vi "gearedMotorPosControl (SubVI).vi"(6 "Reset":bool, 8 "error in (no error)":errorcluster, 9 "PID gains":T1={"proportional gain (Kc)"=2.0, "integral time (Ti, min)"=0.01, "derivative time (Td, min)"=0.00010000000000000003}, 10 "Position (deg)":dbl, 11 "dt":i64) -> (0 "error out":errorcluster, 1 "Waveform Chart":T2(graph), 2 "MotorEncoder (deg)":dbl)   [LabVIEW 2019, in "SJCube.lvlib"]
uses:
  SJCube.lvlib
  <vilib>/addons/control/pid/NI_PID_pid.lvlib
  <vilib>/addons/control/pid/pid.llb/PID (DBL).vi
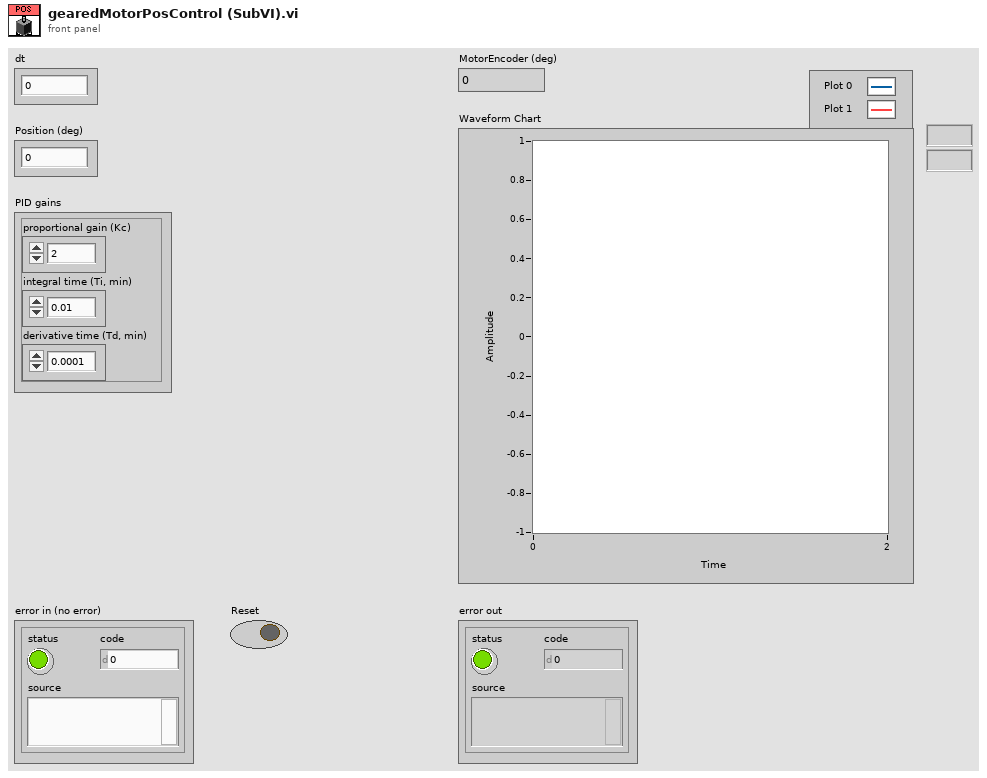
[diagram p1: front panel]
types:
  T1 = cluster{"proportional gain (Kc)":dbl, "integral time (Ti, min)":dbl, "derivative time (Td, min)":dbl}
  T2 = cluster{"Position (deg)":dbl, "MotorEncoder (deg)":dbl}
  T3 = cluster{"Position (deg)":dbl, "gearedMotorEncoder (deg)":dbl}
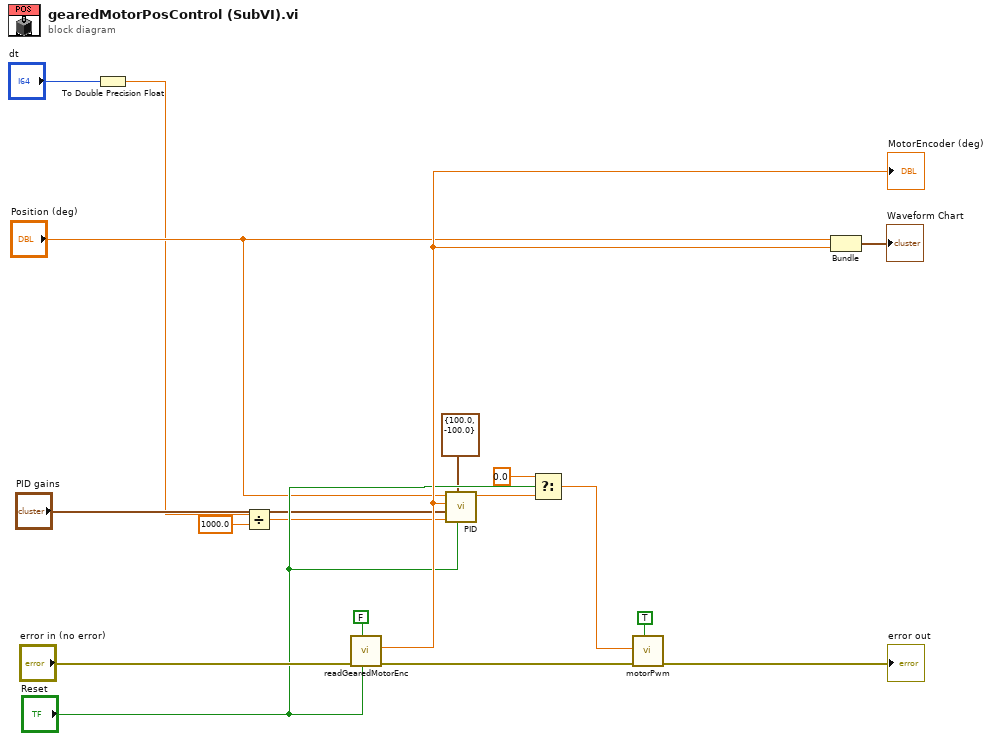
[diagram p0: block diagram]
diagram:
  n1 = To Double Precision Float(number="dt") -> (double precision float=w3:dbl)
  n2 = Divide(x=w3, y=1000.0) -> (x/y=w1:dbl)
  n3 = call "readGearedMotorEnc.vi"("Reset Counter"="Reset", "Reverse ENC?"=FALSE, "error in (no error)"="error in (no error)") -> ("error out"=w10:errorcluster, "gearedMotorEncoder (deg)"=w16:dbl)  [unwired: 7 in]
  "MotorEncoder (deg)" <- w16
  n4 = call-poly <vilib>:"PID.vi"("reinitialize? (F)"="Reset", "output range"=cluster{"output high":dbl, "output low":dbl} {"output high"=100.0, "output low"=-100.0}, "dt (s)"=w1, "PID gains"="PID gains", "process variable"=w16, "setpoint"="Position (deg)") -> ("output"=w14:dbl)  [unwired: 4 in, 1 out]
  n5 = Select(t=0.0, s="Reset", f=w14) -> (s? t:f=w15:dbl)
  n6 = call "motorPwm.vi"("reverse?"=TRUE, "error in (no error)"=w10, "Speed (PWM)"=w15) -> ("error out"=→"error out":errorcluster)  [unwired: 8 in]
  n7 = Bundle("Position (deg)"="Position (deg)", "gearedMotorEncoder (deg)"=w16) -> (→"Waveform Chart":T3)  [unwired: 1 in]
